vi "VariableDeleteUI.vi"(10 "VariableName":string, 11 "VariableManagerRef in":refnum<vi>) -> (3 "VariableManagerRef out":refnum<vi>)   [LabVIEW 2013]
doc: "Create a confirmation window for deleting a variable of the given VariableManager reference."
uses:
  VariableManager/VariableManager.lvclass
  API/VariableManagerAPI.lvlib
panel:
  in  "Cancel":bool
  in  "OK":bool
  out "Display":string
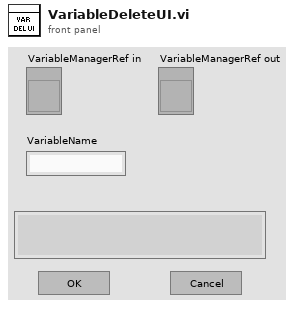
[diagram p1: front panel]
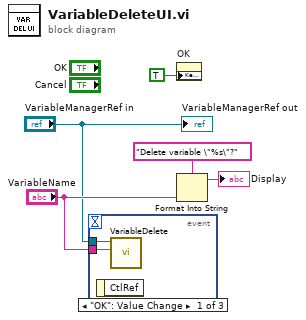
[diagram p0: block diagram]
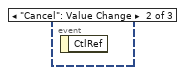
[diagram p2: hidden frame]
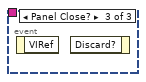
[diagram p3: hidden frame]
diagram:
  n1 = event shown="[0] \"OK\": Value Change" {
    selector: _ -> [_ _ _]
    dyn-events: _ -> [_ _ _]
    timeout: _ -> [_ _ _]
    tunnel: "VariableName" -> [w6 _ _]
    tunnel: "VariableManagerRef in" -> [w7 _ _]
    event "OK": Value Change {
      n2 = event-data() -> ()  [unwired: 1 in, 1 out]
      n3 = call "VariableDelete.vi"("VariableName"=w6, "VariableManagerRef in"=w7) -> ()  [unwired: 8 in, 2 out]
    }
    event "Cancel": Value Change {
      n4 = event-data() -> ()  [unwired: 1 in, 1 out]
    }
    event Panel Close? {
      n5 = event-data() -> ()  [unwired: 1 in, 1 out]
      n6 = event-data() -> ()  [unwired: 2 in, 1 out]
    }
  }
  n7 = property on="OK" class="Bool (strict)"("Key Focus"=TRUE) -> ()  [unwired: 2 in, 2 out]
  n8 = Format Into String(format string="Delete variable \"%s\"?", "VariableName") -> (resulting string=→"Display":string)  [unwired: 2 in, 1 out]
  "VariableManagerRef out" <- "VariableManagerRef in"
